vi "_Persist Entity.vi"(8 "error in (no error)":errorcluster, 9 "Entity":refnum<class "Entity.lvclass">, 10 "Types":refnum<class "Type.lvclass">[](array[class]), 11 "Database in":refnum<class "Database Platform.lvclass">) -> (0 "error out":errorcluster, 3 "Database out":refnum<class "Database Platform.lvclass">)   [LabVIEW 2020, in "Conditum.lvlib" / "Database Platform.lvclass"]
uses:
  Database Platform.lvclass
  Columns/Type/Type.lvclass
  Entity/Entity.lvclass
  Database Platform.lvclass/Database Platform.ctl
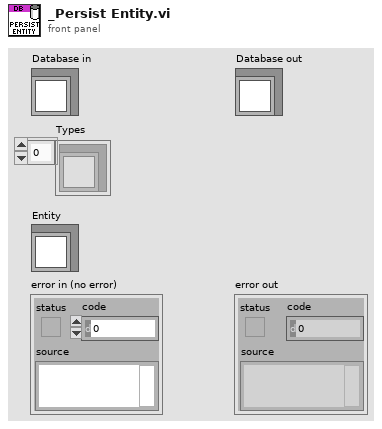
[diagram p1: front panel]
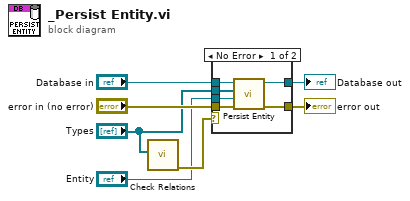
[diagram p0: block diagram]
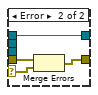
[diagram p2: hidden frame]
diagram:
  n1 = call "Check Relations.vi"("Types"="Types") -> ("error out"=w7:errorcluster)  [unwired: 10 in]
  n2 = case shown="No Error" w7 {
    selector: w7 -> [_ w16]
    tunnel: "Database in" -> [w13 w14]
    tunnel: "error in (no error)" -> [w12 w17]
    tunnel: "Entity" -> [w11 _]
    tunnel: [w10 w15] -> w3
    tunnel: [w9 w14] -> w2
    tunnel: "Types" -> [w8 _]
    frame No Error {
      n3 = call-dynamic "Persist Entity.vi"("error in (no error)"=w12, "Conditum:Entity"=w11, "Types"=w8, "Database in"=w13) -> ("error out"=w10:errorcluster, "Database out"=w9:refnum<class "Database Platform.lvclass">)  [unwired: 6 in]
    }
    frame Error {
      n4 = Merge Errors(w17, w16) -> (w15:errorcluster)
    }
  }
  "error out" <- w3
  "Database out" <- w2
